vi "_Request StringList with lvcsm Support2.vi"(5 "API Ref":refnum<vi>, 6 "Config Path (\"\" For Lvcsm File)":path, 7 "Current Module (\"\" to Generate an ID)":string, 8 "error in (no error)":errorcluster, 9 "Force? (F)":bool, 10 "API Name":string="CSMAPI", 11 "CSM Name":string) -> (0 "error out":errorcluster, 3 "CSMAPI List":string[](array[string]))   [LabVIEW 2017, in "CSM-Helper API with lvcsm Support.lvlib"]
uses:
  CSM-Helper API with lvcsm Support.lvlib
  b7efc127-9b6c-49b9-9e9d-39643bcb625b.vi
  166189b3-b0ee-4f88-bea7-bb947d9812ee.vi
  <vilib>/Utility/config.llb/Close Config Data.vi
  <vilib>/Utility/config.llb/Write Key.vi
  <vilib>/Utility/config.llb/Write Key (Double).vi
  <vilib>/Utility/config.llb/Write Key (I32).vi
  <vilib>/Utility/config.llb/Write Key (String).vi
  lvcsmFile/Path to lvcsm String.vi
  <vilib>/Utility/config.llb/Remove Key.vi
  <vilib>/Utility/config.llb/Get Key Names.vi
  <vilib>/Utility/Data Type/Get Type Information.vi
  <vilib>/Utility/Data Type/Get Array Information.vi
  <vilib>/Utility/config.llb/Write Key (Boolean).vi
  <vilib>/Utility/config.llb/Open Config Data.vi
  lvcsmFile/lvcsm File Path.vi
  lvcsmFile/_Array of VData to VCluster.vi
  <vilib>/Utility/config.llb/Read Key.vi
  <vilib>/Utility/config.llb/Read Key (Double).vi
  <vilib>/Utility/config.llb/Read Key (I32).vi
  lvcsmFile/lvcsm String to Path.vi
  <vilib>/Utility/config.llb/Read Key (String).vi
  <vilib>/Utility/config.llb/Read Key (Boolean).vi
  CSM-Helper.lvclass
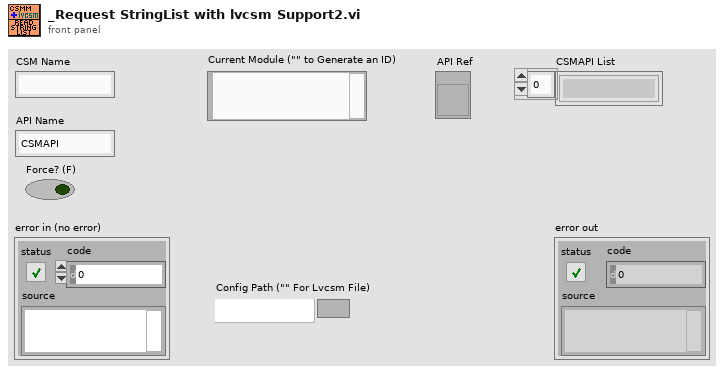
[diagram p1: front panel]
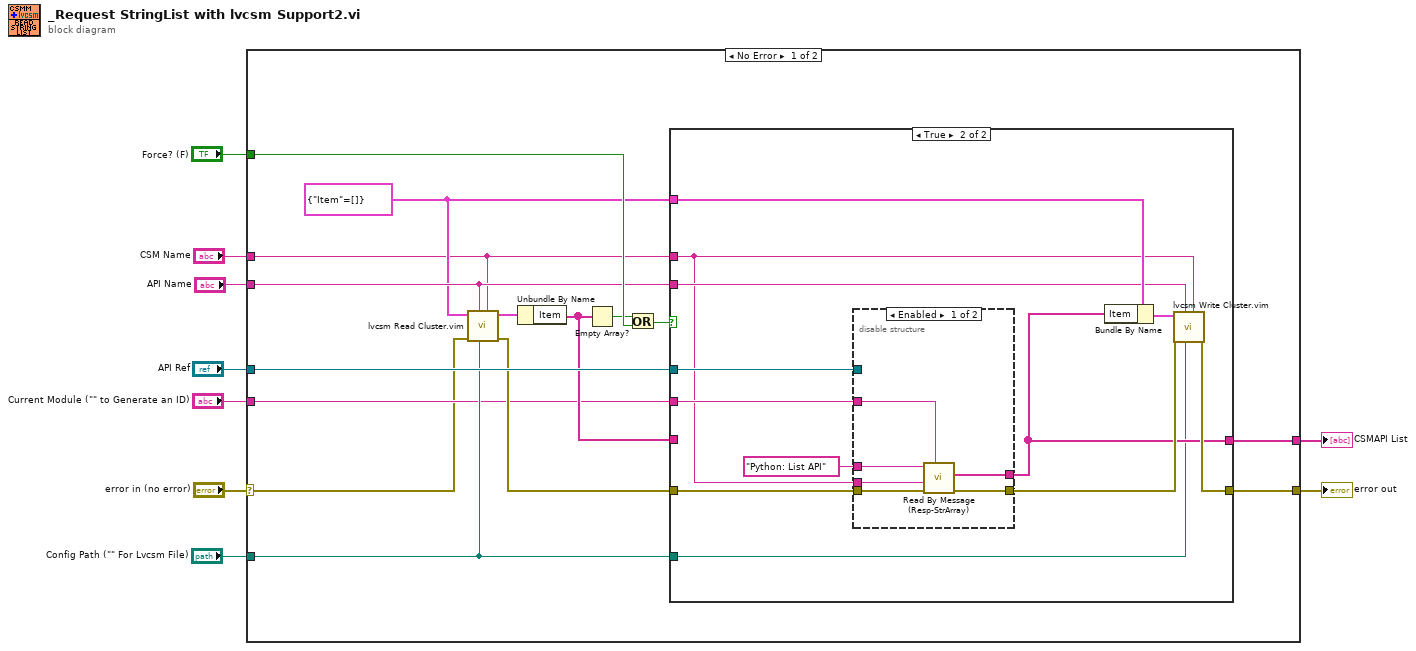
[diagram p0: block diagram]
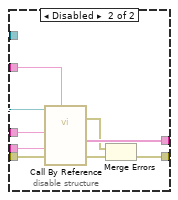
[diagram p3: hidden frame]
diagram:
  n1 = case shown="No Error" "error in (no error)" {
    selector: "error in (no error)" -> [w10 w54]
    tunnel: [w24 w54] -> w9
    tunnel: "CSM Name" -> [w11 _]
    tunnel: "Current Module (\"\" to Generate an ID)" -> [w12 _]
    tunnel: [w23 _] -> w5
    tunnel: "Force? (F)" -> [w22 _]
    tunnel: "Config Path (\"\" For Lvcsm File)" -> [w19 _]
    tunnel: "API Ref" -> [w21 _]
    tunnel: "API Name" -> [w20 _]
    frame No Error {
      w15 = cluster{"Item":string[]} {"Item"=[]}
      n2 = call "lvcsm Read Cluster.vim"("Sub-section (\"\")"=w11, "Config Path"=w19, "Section"=w20, "Error In"=w10, "Default Prototype"=w15) -> ("error out"=w16:errorcluster, "Cluster (Dup)"=w18:cluster{"Item":string[]})  [unwired: 5 in]
      n3 = Unbundle By Name(w18) -> ("Item"=w14:string[])
      n4 = Empty Array?(array=w14) -> (empty?=w17:bool)
      n5 = Or(x=w17, y=w22) -> (x .or. y?=w13:bool)
      n6 = case shown="True" w13 {
        tunnel: w16 -> [w26 w37]
        tunnel: [w26 w34] -> w24
        tunnel: w15 -> [_ w36]
        tunnel: w20 -> [_ w33]
        tunnel: w11 -> [_ w28]
        tunnel: [w25 w32] -> w23
        tunnel: w14 -> [w25 _]
        tunnel: w19 -> [_ w31]
        tunnel: w21 -> [_ w30]
        tunnel: w12 -> [_ w29]
        frame False {
        }
        frame True {
          n7 = disable-structure shown="Enabled" {
            disable-tunnel: [w43 w49] -> w38
            disable-tunnel: w37 -> [w44 w52]
            disable-tunnel: [w42 w50] -> w32
            disable-tunnel: w30 -> [_ w53]
            disable-tunnel: w29 -> [w40 w47]
            disable-tunnel: w28 -> [w41 w46]
            disable-tunnel: "Python: List API" ("State") -> [w39 w45]
            frame Enabled {
              n8 = call "Read By Message (Resp-StrArray).vi"("Current Module (\"\" to Generate an ID)"=w40, "error in (no error)"=w44, "CSM Name"=w41, "State"=w39) -> ("error out"=w43:errorcluster, "Value"=w42:string[])  [unwired: 6 in]
            }
            frame Disabled {
              n9 = call-by-ref "?"(reference=w53, "Current Module (\"\" to Generate an ID)"=w47, "error in (no error)"=w52, "CSM Name"=w46, "State"=w45) -> (error out=w48:errorcluster, 0:"error out"=w51:errorcluster, "Value"=w50:string[])  [unwired: 7 in, 1 out]
              n10 = Merge Errors(w48, w51) -> (w49:errorcluster)
            }
          }
          n11 = Bundle By Name(cluster=w36, "Item"=w32) -> (w35:cluster{"Item":string[]})
          n12 = call "lvcsm Write Cluster.vim"("Sub-section (\"\")"=w28, "Config Path"=w31, "Section"=w33, "Error In"=w38, "Configuration"=w35) -> ("error out"=w34:errorcluster)  [unwired: 6 in]
        }
      }
    }
    frame Error {
    }
  }
  "error out" <- w9
  "CSMAPI List" <- w5
